vi "Get Master and Local Mod IOVs.vi"(8 "error in (no error)":errorcluster, 11 "IOV Engine in":refnum<k21>="ni.var.io:/") -> (0 "error IO":errorcluster, 1 "All Masters":refnum<k21>[](array[refnum]), 2 "All Local Mods":refnum<k21>[](array[refnum]), 3 "Local UDV Container":refnum<k21>[](array[refnum]))   [LabVIEW 2011, in "Scan Engine Custom Device.lvlib"]
uses:
  Scan Engine Custom Device.lvlib
  Program Files (x86)/National Instruments/LabVIEW 2011/resource/objmgr/ni.var.rc
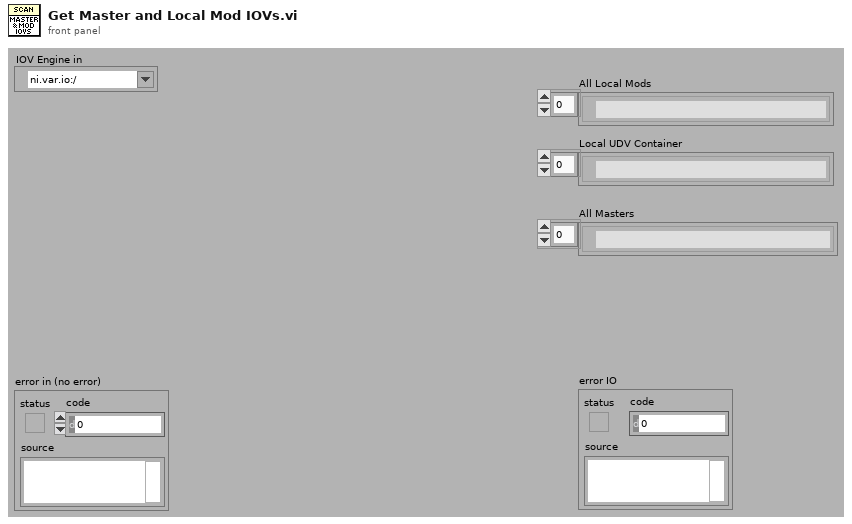
[diagram p1: front panel]
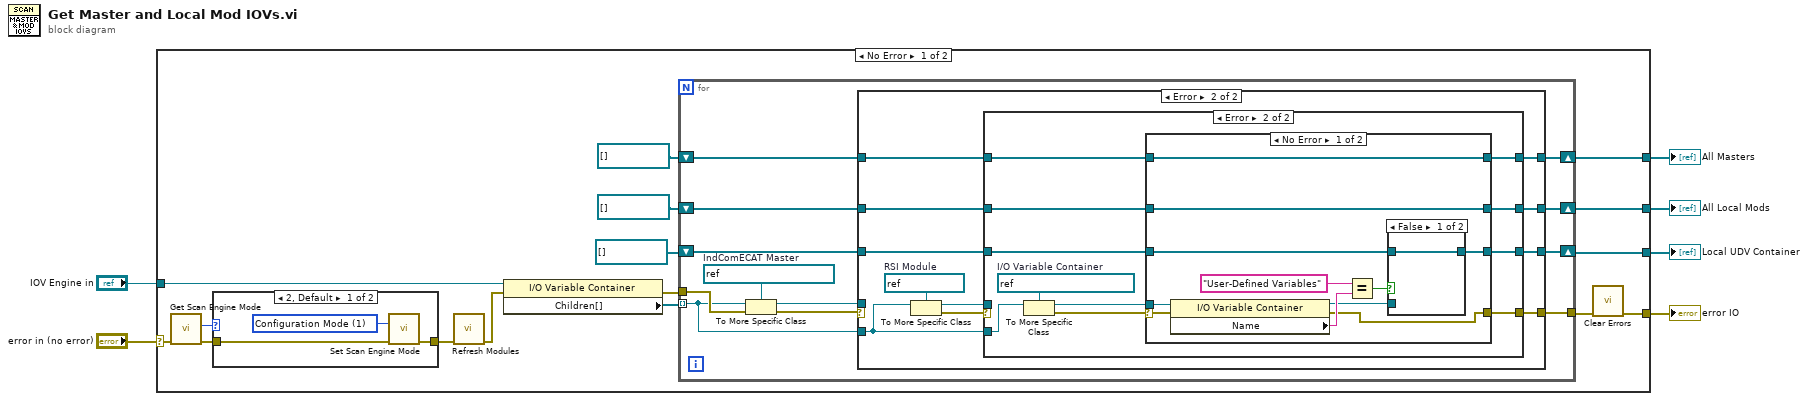
[diagram p0: block diagram]
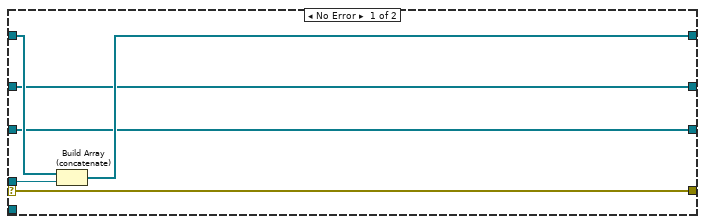
[diagram p3: hidden frame]
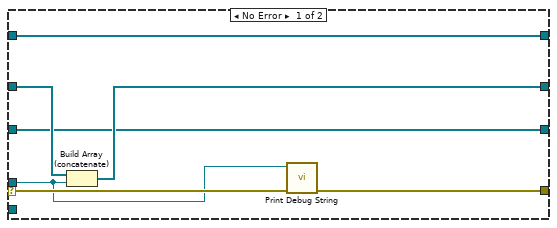
[diagram p4: hidden frame]
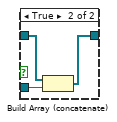
[diagram p5: hidden frame]
diagram:
  n1 = case shown="No Error" "error in (no error)" {
    selector: "error in (no error)" -> [w8 w93]
    tunnel: [w22 w93] -> w6
    tunnel: [w19 _] -> w5
    tunnel: "IOV Engine in" -> [w16 _]
    tunnel: [w14 _] -> w2
    tunnel: [w12 _] -> w1
    frame No Error {
      n2 = call <vilib>:"Get Scan Engine Mode.vi"("error in (no error)"=w8) -> ("error out"=w10:errorcluster, "mode"=w9:i32)  [unwired: 9 in]
      n3 = case shown="2, Default" w9 {
        tunnel: w10 -> [w24 w26]
        tunnel: [w23 w26] -> w11
        frame 2, Default {
          w25 = 1 items=["Configuration Mode"=1, "Active Mode"=2] ("mode (Active Mode)")
          n4 = call <vilib>:"Set Scan Engine Mode.vi"("mode (Active Mode)"=w25, "error in (no error)"=w24) -> ("error out"=w23:errorcluster)  [unwired: 13 in]
        }
        frame 1 {
        }
      }
      n5 = call <vilib>:"Refresh Modules.vi"("error in (no error)"=w11) -> ("error out"=w7:errorcluster)  [unwired: 10 in]
      n6 = property class="I/O Variable Container"(reference=w16, error in=w7) -> (error out=w18:errorcluster, "Children[]"=w17:refnum<k21>[])  [unwired: 1 out]
      n7 = for {
        tunnel: w17 -> [w31] mode=indexing
        tunnel: w18 -> [w38]
        shift-right: [w34] -> w19
        shift-left: refnum<k21>[] [] -> [w33]
        tunnel: [w32] -> w21
        shift-right: [w29] -> w14
        shift-left: refnum<k21>[] [] -> [w30]
        shift-right: [w27] -> w12
        shift-left: refnum<k21>[] [] -> [w28]
        w37 = refnum<k21> refnum  # IndComECAT Master
        n8 = To More Specific Class(target class=w37, reference=w31, error in=w38) -> (specific class reference=w35:refnum<k21>, error out=w36:errorcluster)
        n9 = case shown="Error" w36 {
          selector: w36 -> [w42 _]
          tunnel: w35 -> [w39 _]
          tunnel: [w44 w49] -> w34
          tunnel: w33 -> [w43 w50]
          tunnel: [w42 w48] -> w32
          tunnel: w31 -> [_ w47]
          tunnel: w30 -> [w41 w52]
          tunnel: [w41 w51] -> w29
          tunnel: w28 -> [w40 w46]
          tunnel: [w40 w45] -> w27
          frame No Error {
            n10 = Build Array (concatenate)(w43, w39) -> (w44:refnum<k21>[])
          }
          frame Error {
            w55 = refnum<k21> refnum  # RSI Module
            n11 = To More Specific Class(target class=w55, reference=w47) -> (specific class reference=w53:refnum<k21>, error out=w54:errorcluster)  [unwired: 1 in]
            n12 = case shown="Error" w54 {
              tunnel: w53 -> [w56 _]
              selector: w54 -> [w57 _]
              tunnel: w52 -> [w62 w69]
              tunnel: [w61 w66] -> w51
              tunnel: w50 -> [w60 w68]
              tunnel: [w60 w67] -> w49
              tunnel: [w58 w63] -> w48
              tunnel: w47 -> [_ w72]
              tunnel: w46 -> [w59 w70]
              tunnel: [w59 w65] -> w45
              frame No Error {
                n13 = Build Array (concatenate)(w62, w56) -> (w61:refnum<k21>[])
                n14 = call "Print Debug String.vi"("error in"=w57, "String to write"=w56) -> ("error out"=w58:errorcluster)  [unwired: 8 in]
              }
              frame Error {
                w73 = refnum<k21> refnum  # I/O Variable Container
                n15 = To More Specific Class(target class=w73, reference=w72) -> (specific class reference=w64:refnum<k21>, error out=w71:errorcluster)  [unwired: 1 in]
                n16 = case shown="No Error" w71 {
                  selector: w71 -> [w82 w89]
                  tunnel: w70 -> [w76 w92]
                  tunnel: w69 -> [w83 w91]
                  tunnel: w68 -> [w84 w90]
                  tunnel: [w84 w90] -> w67
                  tunnel: [w83 w91] -> w66
                  tunnel: [w75 w92] -> w65
                  tunnel: w64 -> [w81 _]
                  tunnel: [w74 w89] -> w63
                  frame No Error {
                    n17 = property class="I/O Variable Container"(reference=w81, error in=w82) -> (reference out=w77:refnum<k21>, error out=w74:errorcluster, "Name"=w80:string)
                    n18 = Equal?(x="User-Defined Variables", y=w80) -> (x = y?=w78:bool)
                    n19 = case shown="False" w78 {
                      tunnel: w77 -> [_ w87]
                      tunnel: w76 -> [w85 w88]
                      tunnel: [w85 w86] -> w75
                      frame False {
                      }
                      frame True {
                        n20 = Build Array (concatenate)(w88, w87) -> (w86:refnum<k21>[])
                      }
                    }
                  }
                  frame Error {
                  }
                }
              }
            }
          }
        }
      }
      n21 = call <vilib>:"Clear Errors.vi"("error in (no error)"=w21) -> ("error out"=w22:errorcluster)  [unwired: 6 in]
    }
    frame Error {
    }
  }
  "All Masters" <- w5
  "error IO" <- w6
  "All Local Mods" <- w2
  "Local UDV Container" <- w1
